vi "Data.Build Results Table.vi"(8 "Show Only Failures":bool, 9 "Filter":string, 10 "Attribute Data":T5[](array[typedef]) {"Status" items=["LOG", "PASS", "FAIL", "ERROR"]}, 11 "Numeric Data":T2[](array[typedef]) {"Status" items=["LOG", "PASS", "FAIL", "ERROR"]}) -> (3 "Results Table":T1[](array[typedef]))   [LabVIEW 2024, in "EQMF.lvlib" / "Data.lvlib"]
uses:
  Data.lvlib
  TypeDefs/Data.Result Attribute.ctl
  TypeDefs/Data.Result Item Status.ctl
  TypeDefs/Data.Result Numeric.ctl
  TypeDefs/Data.Result Numeric Limit Type.ctl
  TypeDefs/Data.Result Table Item.ctl
  <vilib>/Utility/error.llb/Trim Whitespace One-Sided.vi
panel:
  # "Step                          Name                                             Value                      Units    LimType        LL            UL          Result           Code                     Description"
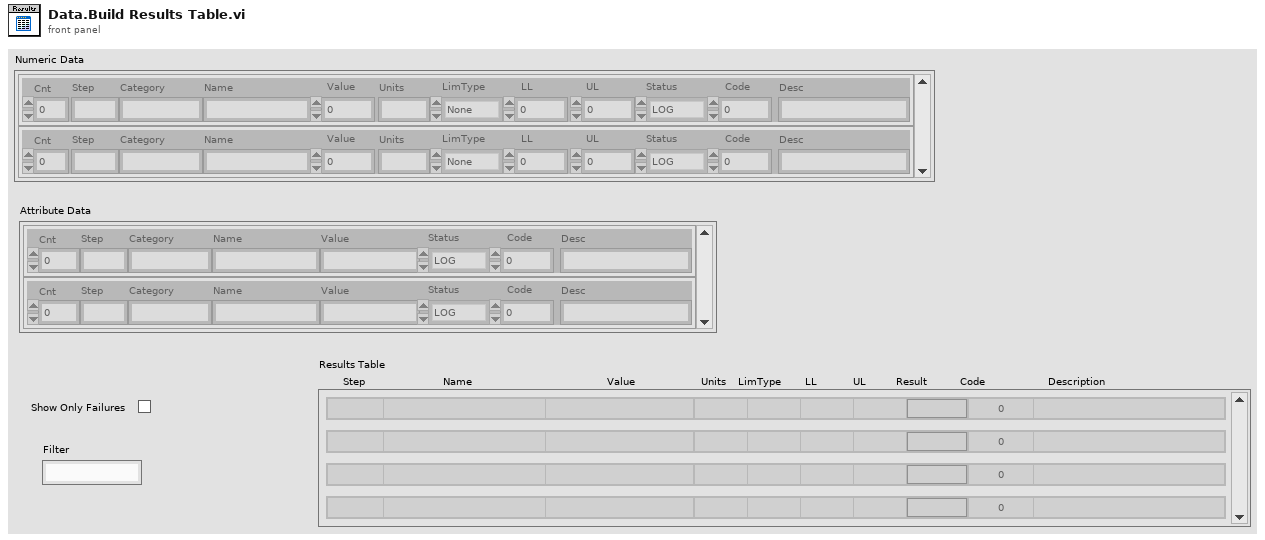
[diagram p1: front panel]
types:
  T1 = typedef "EQMF.lvlib/Data.lvlib/Data.Result Table Item.ctl" = cluster{"Cnt":i32, "Step":string, "Category":string, "Name":string, "Value":string, "Units":string, "LimType":string, "LL":string, "UL":string, "Status":string, "Status Color":u32, "Code":i32, "Desc":string}
  T2 = typedef "EQMF.lvlib/Data.lvlib/Data.Result Numeric.ctl" = cluster{"Cnt":i32, "Step":string, "Category":string, "Name":string, "Value":dbl, "Units":string, "LimType":T3, "LL":dbl, "UL":dbl, "Status":T4, "Code":i32, "Desc":string}
  T3 = typedef "EQMF.lvlib/Data.lvlib/Data.Result Numeric Limit Type.ctl" = enum16{"None", "EQ", "NE", "GT", "LT", "GE", "LE", "GTLT", "GELE", "GELT", "GTLE", "LTGT", "LEGE", "LEGT", "LTGE"}
  T4 = typedef "EQMF.lvlib/Data.lvlib/Data.Result Item Status.ctl" = i32
  T5 = typedef "EQMF.lvlib/Data.lvlib/Data.Result Attribute.ctl" = cluster{"Cnt":i32, "Step":string, "Category":string, "Name":string, "Value":string, "Status":T4, "Code":i32, "Desc":string}
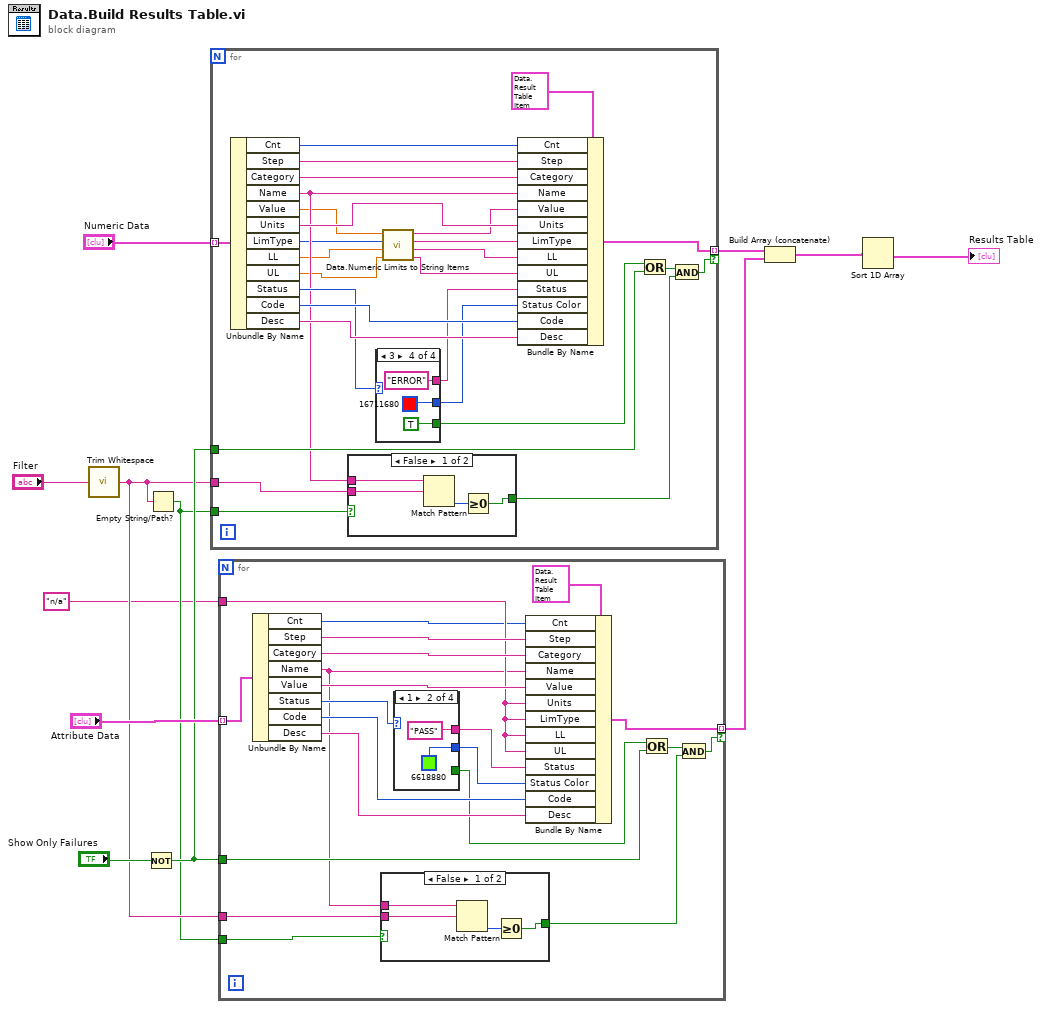
[diagram p0: block diagram]
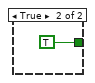
[diagram p2: hidden frame]
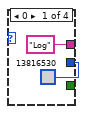
[diagram p3: hidden frame]
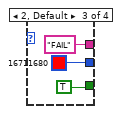
[diagram p4: hidden frame]
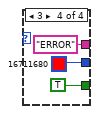
[diagram p5: hidden frame]
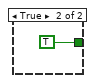
[diagram p6: hidden frame]
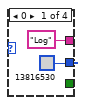
[diagram p7: hidden frame]
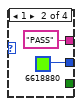
[diagram p8: hidden frame]
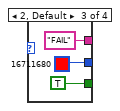
[diagram p9: hidden frame]
diagram:
  n1 = call <vilib>:"Trim Whitespace.vi"("string"="Filter") -> ("trimmed string"=w4:string)  [unwired: 1 in]
  n2 = Not(x="Show Only Failures") -> (.not. x?=w6:bool)
  n3 = Empty String/Path?(string/path=w4) -> (empty?=w3:bool)
  n4 = for {
    tunnel: "Numeric Data" -> [w39] mode=indexing
    tunnel: [w33] -> w11 mode=indexing if=w23
    tunnel: w6 -> [w27]
    tunnel: w4 -> [w25]
    tunnel: w3 -> [w21]
    n5 = Unbundle By Name(w39) -> ("Cnt"=w29:i32, "Step"=w38:string, "Category"=w37:string, "Name"=w26:string, "Value"=w18:dbl, "Units"=w34:string, "LimType"=w20:T3, "LL"=w17:dbl, "UL"=w16:dbl, "Status"=w32:T4, "Code"=w35:i32, "Desc"=w36:string)
    n6 = case shown="False" w21 {
      tunnel: w25 -> [w44 _]
      tunnel: w26 -> [w43 _]
      tunnel: [w41 TRUE] -> w22
      frame False {
        n7 = Match Pattern(string=w43, regular expression=w44) -> (offset past match=w42:i32)  [unwired: 1 in, 3 out]
        n8 = Greater Or Equal To 0?(x=w42) -> (x >= 0?=w41:bool)
      }
      frame True {
      }
    }
    n9 = case shown="3" w32 {
      tunnel: [u32 13816530 u32 6618880 u32 16711680 u32 16711680] -> w30
      tunnel: ["Log" "PASS" "FAIL" "ERROR"] -> w31
      tunnel: [_ _ TRUE TRUE] -> w28
      frame 0 {
      }
      frame 1 {
      }
      frame 2, Default {
      }
      frame 3 {
      }
    }
    n10 = call "Data.Numeric Limits to String Items.vi"("UL"=w16, "LL"=w17, "LimType"=w20, "Value"=w18) -> ("UL"=w15:string, "LL"=w14:string, "LimType"=w19:string, "Value"=w13:string)  [unwired: 4 in]
    n11 = Bundle By Name(cluster=T1 {"Cnt"=0, "Step"="", "Category"="", "Name"="", "Value"="", "Units"="", "LimType"="", "LL"="", "UL"="", "Status"="", "Status Color"=16448250, "Code"=0, "Desc"=""} ("Result Item"), "Cnt"=w29, "Step"=w38, "Category"=w37, "Name"=w26, "Value"=w13, "Units"=w34, "LimType"=w19, "LL"=w14, "UL"=w15, "Status"=w31, "Status Color"=w30, "Code"=w35, "Desc"=w36) -> (w33:T1)
    n12 = Or(x=w28, y=w27) -> (x .or. y?=w24:bool)
    n13 = And(x=w24, y=w22) -> (x .and. y?=w23:bool)
  }
  n14 = for {
    tunnel: "Attribute Data" -> [w76] mode=indexing
    tunnel: [w71] -> w10 mode=indexing if=w61
    tunnel: "n/a" ("N/A Filler") -> [w67]
    tunnel: w6 -> [w64]
    tunnel: w4 -> [w58]
    tunnel: w3 -> [w57]
    n15 = Unbundle By Name(w76) -> ("Cnt"=w65:i32, "Step"=w75:string, "Category"=w74:string, "Name"=w59:string, "Value"=w68:string, "Status"=w70:T4, "Code"=w72:i32, "Desc"=w73:string)
    n16 = case shown="False" w57 {
      tunnel: w58 -> [w80 _]
      tunnel: w59 -> [w79 _]
      tunnel: [w77 TRUE] -> w60
      frame False {
        n17 = Match Pattern(string=w79, regular expression=w80) -> (offset past match=w78:i32)  [unwired: 1 in, 3 out]
        n18 = Greater Or Equal To 0?(x=w78) -> (x >= 0?=w77:bool)
      }
      frame True {
      }
    }
    n19 = case shown="1" w70 {
      tunnel: [u32 13816530 u32 6618880 u32 16711680 u32 16711680] -> w69
      tunnel: ["Log" "PASS" "FAIL" "ERROR"] -> w66
      tunnel: [_ _ TRUE TRUE] -> w63
      frame 0 {
      }
      frame 1 {
      }
      frame 2, Default {
      }
      frame 3 {
      }
    }
    n20 = Bundle By Name(cluster=T1 {"Cnt"=0, "Step"="", "Category"="", "Name"="", "Value"="", "Units"="", "LimType"="", "LL"="", "UL"="", "Status"="", "Status Color"=16448250, "Code"=0, "Desc"=""} ("Result Item"), "Cnt"=w65, "Step"=w75, "Category"=w74, "Name"=w59, "Value"=w68, "Units"=w67, "LimType"=w67, "LL"=w67, "UL"=w67, "Status"=w66, "Status Color"=w69, "Code"=w72, "Desc"=w73) -> (w71:T1)
    n21 = Or(x=w63, y=w64) -> (x .or. y?=w62:bool)
    n22 = And(x=w62, y=w60) -> (x .and. y?=w61:bool)
  }
  n23 = Build Array (concatenate)(w11, w10) -> (w8:T1[])
  n24 = Sort 1D Array(array=w8) -> (sorted array=→"Results Table":T1[])
